vi "AddCustomData.vi"(8 "error in":errorcluster, 11 "SequenceRunReference in":refnum<class "SequenceRunReference.lvclass">) -> (0 "error out":errorcluster, 2 "CustomData":refnum<class "CustomData.lvclass">, 3 "SequenceRunReference out":refnum<class "SequenceRunReference.lvclass">)   [LabVIEW 2021, in "ProligentXMLGenerator.lvlib" / "SequenceRunReference.lvclass"]
doc: "Add a custom data element.\n\nThe values defined under this element will not be interpreted by the DIT. It can be used to store data that will be used by another system."
uses:
  SequenceRunReference.lvclass
  SequenceRunReference.lvclass/SequenceRunReference.ctl
  Model/CustomData/CustomData.lvclass
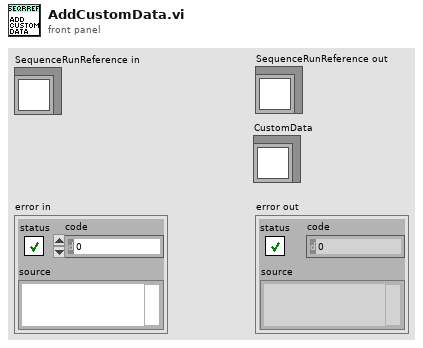
[diagram p1: front panel]
types:
  T1 = typedef "ProligentXMLGenerator.lvlib/SequenceRunReference.lvclass/Data.ctl" = cluster{"Name":string, "CustomData":refnum<class "CustomData.lvclass">, "Id":refnum<class "Guid.lvclass">}
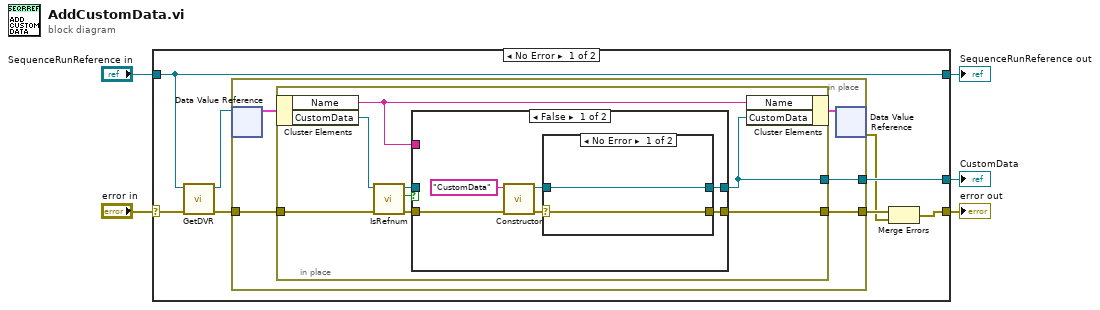
[diagram p0: block diagram]
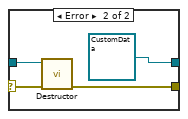
[diagram p2: hidden frame]
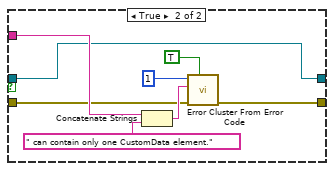
[diagram p3: hidden frame]
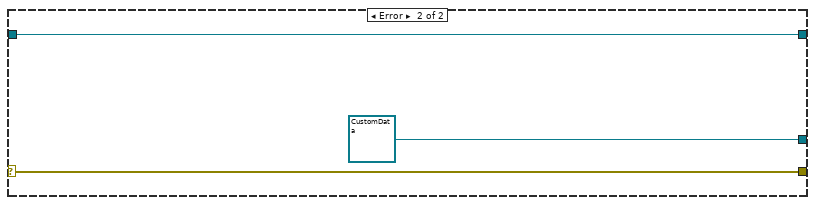
[diagram p4: hidden frame]
diagram:
  n1 = case shown="No Error" "error in" {
    selector: "error in" -> [w11 w48]
    tunnel: [w12 refnum<class "CustomData.lvclass"> refnum ("ProligentResultProcessor:CustomData")] -> w5
    tunnel: [w8 w48] -> w3
    tunnel: "SequenceRunReference in" -> [w6 w49]
    tunnel: [w6 w49] -> w1
    frame No Error {
      n2 = call "GetDVR.vi"("error in"=w11, "SequenceRunReference in"=w6) -> ("error out"=w10:errorcluster, "DVRReference"=w9:refnum<data-value>)  [unwired: 8 in]
      n3 = in-place "In Place Element Structure" {
        in-place-border: [w16] -> w13
        in-place-border: [w17] -> w12
        in-place-border: w10 -> [w18]
        n4 = in-place-dvr #1(w9) -> (w15:T1)  [unwired: 1 out]
        n5 = in-place "In Place Element Structure" {
          in-place-border: w18 -> [w25]
          in-place-border: [w19] -> w17
          in-place-border: [w22] -> w16
          n6 = in-place-cluster #2(w15) -> ("Name"=w20:string, "CustomData"=w21:refnum<class "CustomData.lvclass">)
          n7 = call "IsRefnum.vi"("error in"=w25, "CustomDataType in"=w21) -> ("error out"=w24:errorcluster, "IsRefnum"=w23:bool, "CustomDataType out"=w26:refnum<class "CustomData.lvclass">)  [unwired: 7 in]
          n8 = case shown="False" w23 {
            tunnel: w26 -> [_ w39]
            tunnel: w24 -> [w32 w41]
            tunnel: [w29 w40] -> w22
            tunnel: [w28 w39] -> w19
            tunnel: w20 -> [_ w42]
            frame False {
              n9 = call "Constructor.vi"("error in"=w32, "Name"="CustomData") -> ("error out"=w31:errorcluster, "CustomDataType"=w30:refnum<class "CustomData.lvclass">)  [unwired: 8 in]
              n10 = case shown="No Error" w31 {
                selector: w31 -> [w33 w38]
                tunnel: w30 -> [w34 w36]
                tunnel: [w33 w37] -> w29
                tunnel: [w34 refnum<class "CustomData.lvclass"> refnum ("ProligentResultProcessor:CustomData")] -> w28
                frame No Error {
                }
                frame Error {
                  n11 = call "Destructor.vi"("error in"=w38, "CustomDataType"=w36) -> ("error out"=w37:errorcluster)  [unwired: 9 in]
                }
              }
            }
            frame True {
              n12 = Concatenate Strings(w42, " can contain only one CustomData element." ("string")) -> (w46:string)
              n13 = call <vilib>:"Error Cluster From Error Code.vi"("show call chain? (False)"=TRUE, "error in (no error)"=w41, "error message (\"\")"=w46, "error code (0)"=1) -> ("error out"=w40:errorcluster)  [unwired: 5 in]
            }
          }
          n14 = in-place-cluster #2("Name"=w20, "CustomData"=w19) -> (w14:T1)
        }
        n15 = in-place-dvr #1(w14) -> (w7:errorcluster)  [unwired: 1 out]
      }
      n16 = Merge Errors(w13, w7) -> (w8:errorcluster)
    }
    frame Error {
    }
  }
  "error out" <- w3
  "SequenceRunReference out" <- w1
  "CustomData" <- w5
